vi "QRCodes.vi"(4 "WiFi Info":T4={"WiFi"={"SSID"="", "Key"=""}, "SystemLink"={"APIKey"="", "Tag"="", "Type"="STRING"}}, 5 "ROI":T3, 6 "Output":enum16{"None", "UART", "SPI", "I2C", "WiFi"}(ring), 7 "Camera Setup":T1={"Format"=enum."RGB565", "size"=enum."QVGA (320x240)", "Skip frames (ms)"=2000, "autoGain"=FALSE, "autoWhitebal"=FALSE}, 8 "error in (no error)":errorcluster, 10 "Value":T2(ring), 11 "VISA Refnum in":refnum<visa-resource-name>) -> (0 "error out":errorcluster, 2 "Python Code":string, 3 "VISA Refnum out":refnum<visa-resource-name>)   [LabVIEW 2020]
uses:
  _subs/CameraSetup.ctl
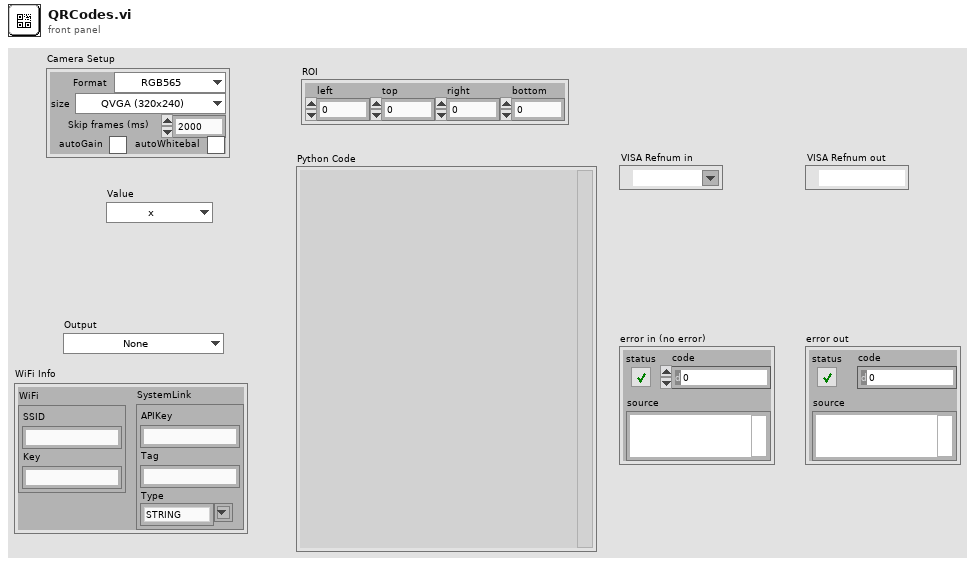
[diagram p1: front panel]
types:
  T1 = typedef "CameraSetup.ctl" = cluster{"Format":enum16{"GRAYSCALE", "RGB565", "BAYER"}, "size":enum16{"QQQQVGA (40x30)", "QQQVGA (80x60)", "QQVGA (160x120)", "QVGA (320x240)", "VGA (640x480)", "LCD (128x160)", "B64x32 (64x32)", "B64x64", "B128x64", "B128x128"}, "Skip frames (ms)":u16, "autoGain":bool, "autoWhitebal":bool}
  T2 = enum16{"x", "y", "w", "h", "payload", "version", "ecc_level", "mask", "data_type", "All data"}
  T3 = cluster{"left":i32, "top":i32, "right":i32, "bottom":i32}
  T4 = cluster{"WiFi":cluster{"SSID":string, "Key":string}, "SystemLink":cluster{"APIKey":string, "Tag":string, "Type":string}}
  T5 = typedef "PythonCtrl.ctl" = cluster{"session":refnum<k35>, "PyPath":path, "Processor":T6}
  T6 = typedef "Processors.ctl" = enum16{"SPIKE", "Pi", "Pi_ssh", "OpenMV"}
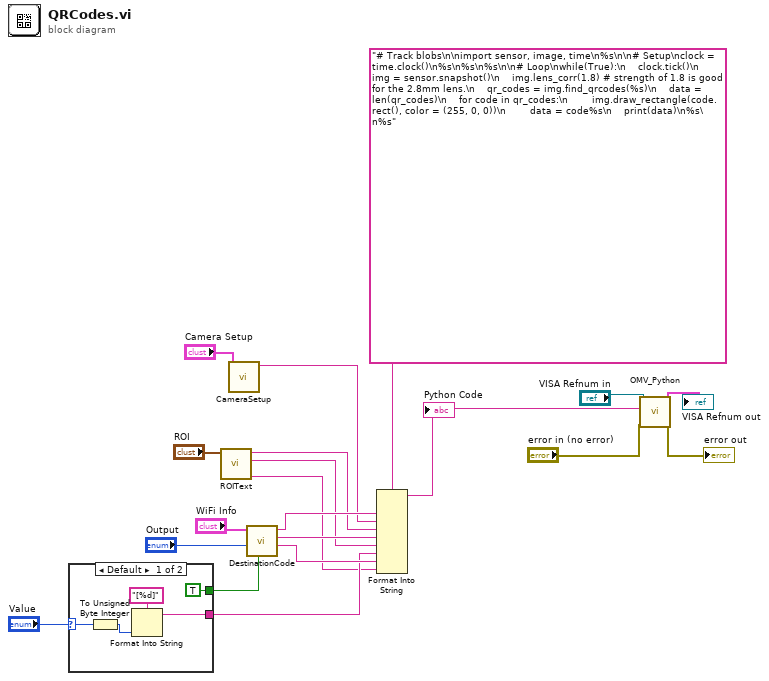
[diagram p0: block diagram]
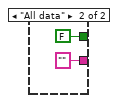
[diagram p2: hidden frame]
diagram:
  n1 = case shown="Default" "Value" {
    selector: "Value" -> [w23 _]
    tunnel: [w24 ""] -> w6
    tunnel: [TRUE FALSE] -> w1
    frame Default {
      n2 = To Unsigned Byte Integer(number=w23) -> (unsigned 8bit integer=w21:u8)
      n3 = Format Into String(format string="[%d]", w21) -> (resulting string=w24:string)  [unwired: 2 in, 1 out]
    }
    frame "All data" {
    }
  }
  n4 = call "ROIText.vi"("ROI"="ROI") -> ("draw"=w2:string, "roi = r"=w3:string, "r"=w4:string)  [unwired: 7 in, 1 out]
  n5 = call "CameraSetup.vi"("Camera Setup"="Camera Setup") -> ("String"=w14:string)  [unwired: 10 in]
  n6 = call "DestinationCode.vi"("Single number?"=w1, "Destination"="Output", "WiFi Info"="WiFi Info") -> ("Repeated call"=w17:string, "Setup"=w18:string, "Headers"=w15:string)  [unwired: 6 in]
  n7 = Format Into String(format string="# Track blobs\n\nimport sensor, image, time\n%s\n\n# Setup\nclock = time.clock()\n%s\n%s\n%s\n\n# Loop\nwhile(True):\n    clock.tick()\n    img = sensor.snapshot()\n    img.lens_corr(1.8) # strength of 1.8 is good for the 2.8mm lens.\n    qr_codes = img.find_qrcodes(%s)\n    data = len(qr_codes)\n    for code in qr_codes:\n        img.draw_rectangle(code.rect(), color = (255, 0, 0))\n        data = code%s\n    print(data)\n%s\n%s" ("startCode"), w15, w14, w4, w18, w3, w6, w17, w2) -> (resulting string=w8:string)  [unwired: 2 in, 1 out]
  "Python Code" <- w8
  n8 = call "OMV_Python.vi"("error in (no error)"="error in (no error)", "Script"=w8, "Python"="VISA Refnum in") -> ("error out"=→"error out":errorcluster, "Python"=→"VISA Refnum out":T5)  [unwired: 7 in]
